vi "HG00_subvi_LPS.vi"(0 "Shift":dbl, 1 "Tilt":dbl[](array[numeric]), 3 "w":dbl, 4 "l":dbl, 5 "Gap":dbl) -> (2 "return value 2":dbl[](array[numeric]))   [LabVIEW 2019]
panel:
  out "Py Script":string
  in  "Array in":dbl[](array[numeric])
  out "error out":errorcluster
  in  "Python version":string="3.6"
  in  "function name":string="lps"
  in  "module path":path=path "C:/Users/edwar/OneDrive/Documents/GitHub/Python-HG-Modes/HG Modes/HG00.py"
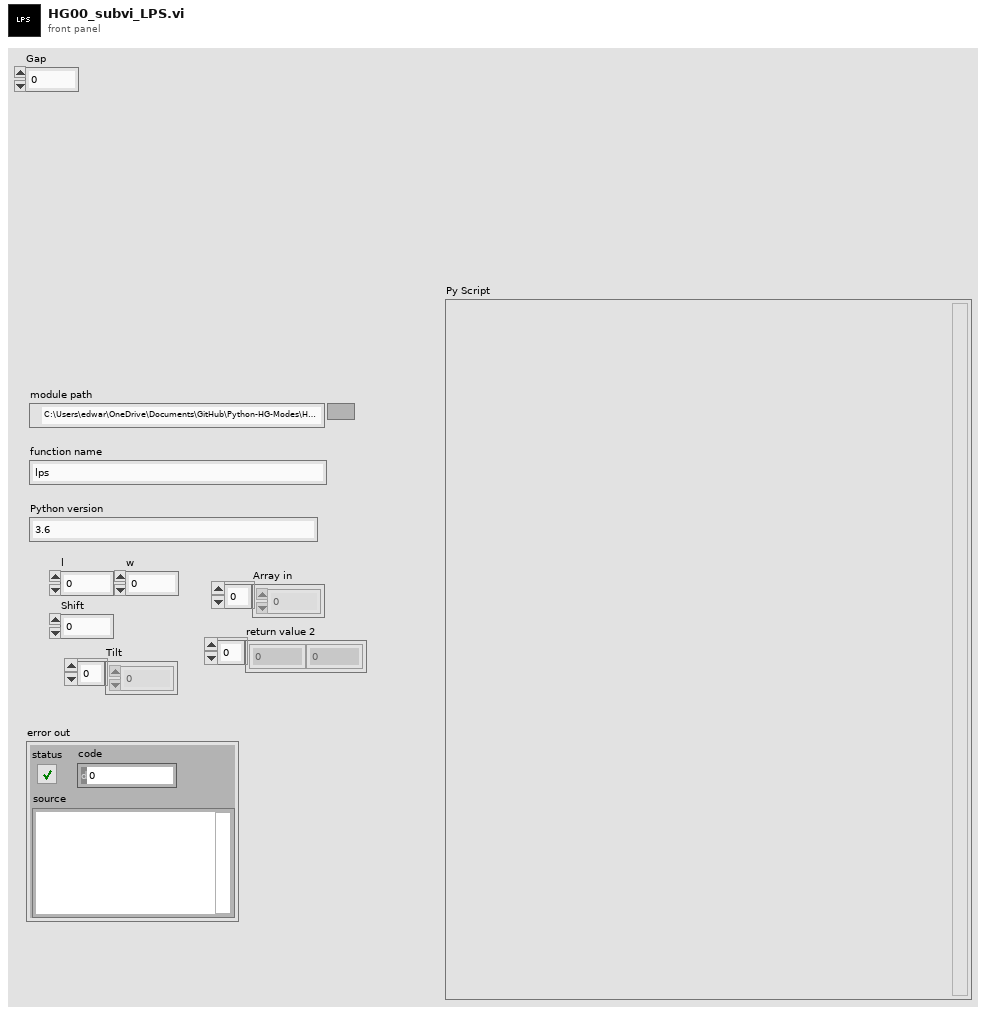
[diagram p1: front panel]
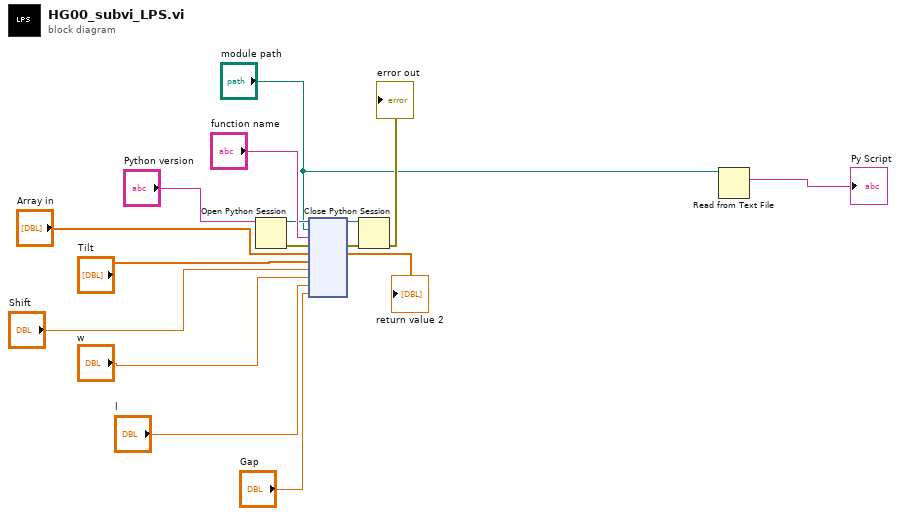
[diagram p0: block diagram]
diagram:
  n1 = Open Python Session(python version="Python version") -> (session out=w5:refnum<k35>, error out=w8:errorcluster)  [unwired: 2 in]
  n2 = node(w5, "module path", "function name", w8, "Array in", "Tilt", "Shift", "w", "l", "Gap") -> (w6:refnum<k35>, w9:errorcluster, →"return value 2":dbl[])  [unwired: 5 in, 2 out]
  "error out" <- w9
  n3 = Close Python Session(session in=w6, error in=w9) -> ()  [unwired: 1 out]
  n4 = Read from Text File(file (use dialog)="module path") -> (text=→"Py Script":string)  [unwired: 3 in, 3 out]
